vi "half adder SubVI).vi"(2 "a":bool, 3 "b":bool) -> (0 "sum":bool, 1 "cout":bool)   [LabVIEW 2012]
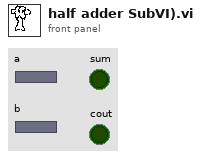
[diagram p1: front panel]
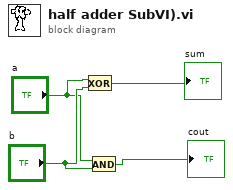
[diagram p0: block diagram]
diagram:
  n1 = Exclusive Or(1:"b", 2:"a") -> (0:→"sum":bool)
  n2 = And(x="a", y="b") -> (x .and. y?=→"cout":bool)
